vi "Test D2XX.vi"() -> ()   [LabVIEW 2019, in "D2XX-lv.lvlib"]
uses:
  D2XX-lv.lvlib
  API/Open Device (index).vi
  <instrlib>/_D2XX/D2XX/FT_Open_Device_By_Index.vi
  <instrlib>/_D2XX/D2XX/D2XX.lvlib
panel:
  out "Device Info Node":T1 {"FT_Handle" format="%.0x"; "LocID" format="%.0x"; "PID" format="%.0x"; "VID" format="%.0x"; "Type" items=["FT232B-FT245B", "FT8U232AM-FT8U245AM", "FT8U100AX", "UNKNOWN", "FT2232", "FT232R", "FT2232H", "FT4232H", "FT232H"]}
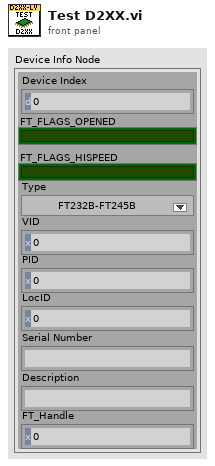
[diagram p1: front panel]
types:
  T1 = cluster{"Device Index":u32, "FT_FLAGS_OPENED":bool, "FT_FLAGS_HISPEED":bool, "Type":u32, "VID":u32, "PID":u32, "LocID":i32, "Serial Number":string, "Description":string, "FT_Handle":u32}
  T2 = cluster{"Device Index":u32, "FT_FLAGS_OPENED":bool, "FT_FLAGS_HISPEED":bool, "Type":u32, "VID":u32, "PID":u32, "LocID":i32, "Serial Number":string, "Description":string, "FT_Handle":u64}
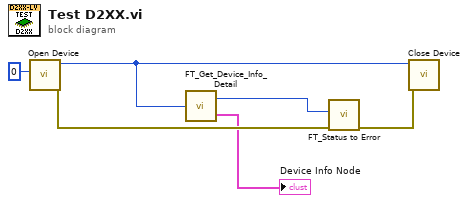
[diagram p0: block diagram]
diagram:
  n1 = call-poly "Open Device.vi"("Device Index"=0) -> ("error out"=w6:errorcluster, "Handle"=w3:u64)  [unwired: 9 in]
  n2 = call <instrlib>:"FT_Get_Device_Info_Detail.vi"("Device Index"=w3) -> ("FT_Status"=w2:u32, "Device Info Node"=→"Device Info Node":T2)
  n3 = call "FT_Status to Error.vi"("error in (no error)"=w6, "FT_Status"=w2) -> ("error out"=w5:errorcluster)  [unwired: 9 in]
  n4 = call "Close Device.vi"("error in (no error)"=w5, "Handle"=w3) -> ()  [unwired: 9 in, 1 out]
